vi "generateUploadZip.vi"(0 "textRef":refnum<vi>, 1 "xmlPath":path=path "d:/bb.ini", 2 "uploadPara":T1, 3 "SN":string, 4 "pnType":string, 5 "error in (no error)":errorcluster) -> (19 "错误输出":errorcluster)   [LabVIEW 2011]
uses:
  dataType/UploadPara.ctl
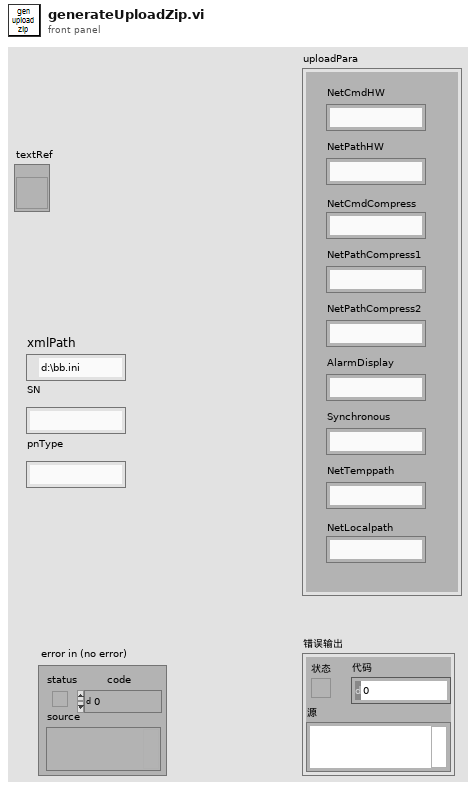
[diagram p1: front panel]
types:
  T1 = typedef "UploadPara.ctl" = cluster{"NetCmdHW":string, "NetPathHW":string, "NetCmdCompress":string, "NetPathCompress1":string, "NetPathCompress2":string, "AlarmDisplay":string, "Synchronous":string, "NetTemppath":string, "NetLocalpath":string}
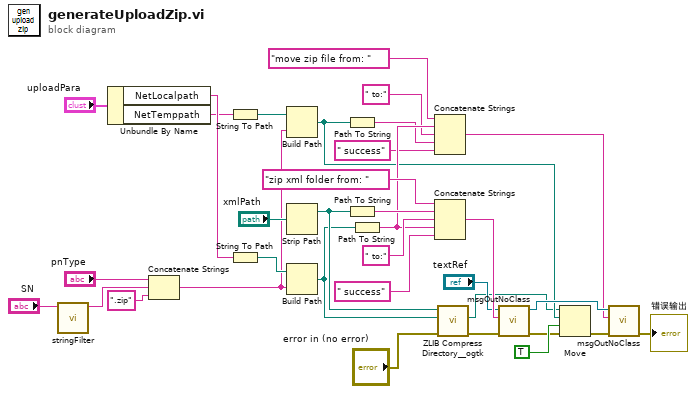
[diagram p0: block diagram]
diagram:
  n1 = call "stringFilter.vi"("stringIn"="SN") -> ("stringOut"=w30:string)  [unwired: 10 in]
  n2 = Unbundle By Name("uploadPara") -> ("NetLocalpath"=w31:string, "NetTemppath"=w26:string)
  n3 = Concatenate Strings("pnType", w30, ".zip" ("字符串")) -> (w24:string)
  n4 = String To Path(string=w26) -> (path=w25:path)
  n5 = String To Path(string=w31) -> (path=w27:path)
  n6 = Build Path(base path=w25, name or relative path=w24) -> (appended path=w8:path)
  n7 = Strip Path(path="xmlPath") -> (stripped path=w17:path)  [unwired: 1 out]
  n8 = Build Path(base path=w27, name or relative path=w24) -> (appended path=w14:path)
  n9 = Path To String(path=w8) -> (string=w7:string)
  n10 = Path To String(path=w17) -> (string=w16:string)
  n11 = Path To String(path=w14) -> (string=w10:string)
  n12 = Concatenate Strings("move zip file from: ", w10, " to:" ("字符串"), w7, " success" ("字符串")) -> (w5:string)
  n13 = Concatenate Strings("zip xml folder from: ", w16, " to:" ("字符串"), w10, " success" ("字符串")) -> (w12:string)
  n14 = call <userlib>:"ZLIB Compress Directory__ogtk.vi"("error in (no error)"="error in (no error)", "archive name (root directory with .zip ending)"=w14, "root directory (file dialog)"=w17) -> ("error out"=w22:errorcluster, "archive name out"=w1:path)  [unwired: 6 in, 1 out]
  n15 = call "msgOutNoClass.vi"("错误输入（无错误）"=w22, "字符串"=w12, "textRef"="textRef") -> ("错误输出"=w21:errorcluster, "引用输出"=w19:refnum<vi>)  [unwired: 7 in]
  n16 = Move(source path=w1, error in=w21, 9:TRUE ("覆盖(F)"), 10:w8) -> (error out=w20:errorcluster)  [unwired: 1 in, 2 out]
  n17 = call "msgOutNoClass.vi"("错误输入（无错误）"=w20, "字符串"=w5, "textRef"=w19) -> ("错误输出"=→"错误输出":errorcluster)  [unwired: 7 in, 1 out]
